vi "user.vi"() -> ()   [LabVIEW 2020]
uses:
  <userlib>/Zaphiro/GTools/Redis/Sources/Redis/Redis.lvclass/Redis.ctl
  aea59807-97c7-47ab-b578-198c3bfad1a9.vi
  f854457d-36a3-4227-beff-9843280818cc.vi
  <userlib>/Zaphiro/GTools/Redis/Sources/Redis/Connection/PING.vi
  aea59807-97c7-47ab-b578-198c3bfad1a9.vi/7c7783df-fd5a-49d9-9b7a-63cc9fb0e4e5.vi
  <userlib>/Zaphiro/GTools/Redis/Sources/Redis/Connection/QUIT.vi
  <userlib>/Zaphiro/GTools/Redis/Sources/Redis/subVIs/LL_collect-response.vi
  <userlib>/Zaphiro/GTools/Redis/Sources/Redis/Redis.lvclass
  b567c38f-e722-4316-83bf-2d80707c7bfa.vi
panel:
  out "ts":string[](array[string])
  in  "check-ts":bool
  out "meas":string[](array[string])
  in  "check-list":bool
  in  "connection":cluster{"ip":string, "port":u16, "timeout":i32}={"ip"="localhost", "port"=6379, "timeout"=1000}
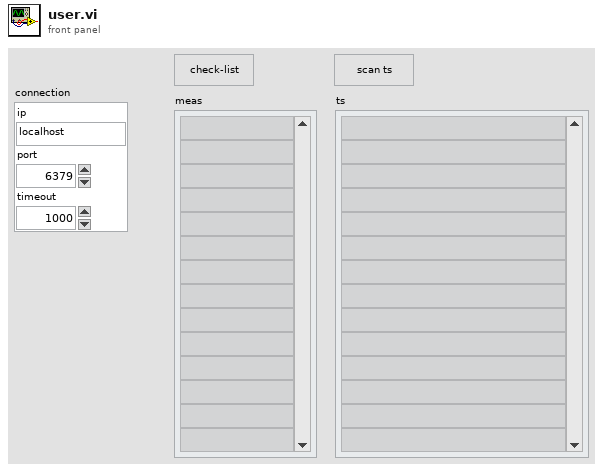
[diagram p1: front panel]
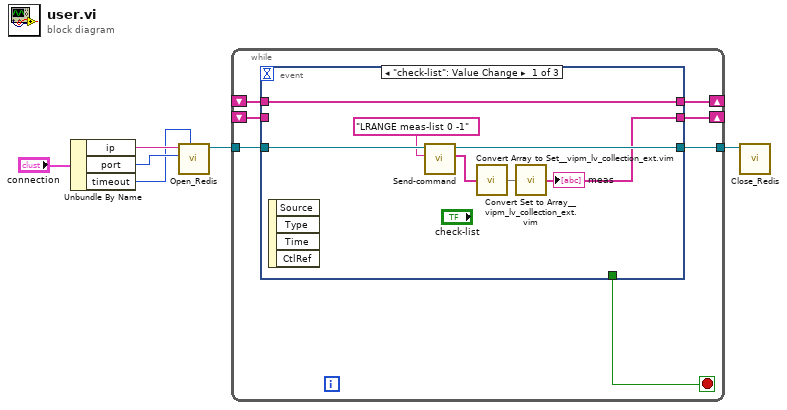
[diagram p0: block diagram]
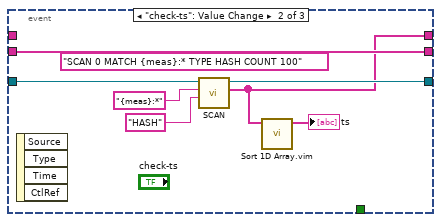
[diagram p2: hidden frame]
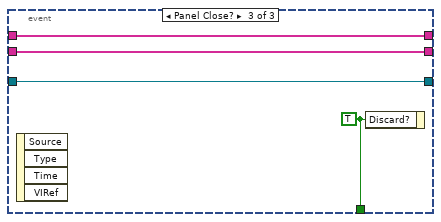
[diagram p3: hidden frame]
diagram:
  n1 = Unbundle By Name("connection") -> ("ip"=w5:string, "port"=w4:u16, "timeout"=w3:i32)
  n2 = call <userlib>:"Open_Redis.vi"("Tcp timeout ms"=w3, "Port"=w4, "Host"=w5) -> ("output cluster"=w2:refnum<class "Redis.lvclass">)  [unwired: 6 in, 2 out]
  n3 = while {
    tunnel: w2 -> [w13]
    tunnel: [w12] -> w1
    shift-right: [w10] -> _
    shift-left: _ -> [w9]
    shift-right: [w8] -> _
    shift-left: _ -> [w7]
    stop <- w11 stop-if-true
    n4 = event shown="[0] \"check-list\": Value Change" {
      selector: _ -> [_ _ _]
      dyn-events: _ -> [_ _ _]
      timeout: _ -> [_ _ _]
      tunnel: w13 -> [w20 w26 w30]
      tunnel: [w19 w25 w30] -> w12
      tunnel: [_ _ w31] -> w11
      tunnel: [w15 w27 w29] -> w10
      tunnel: w9 -> [_ w27 w29]
      tunnel: [w14 w24 w28] -> w8
      tunnel: w7 -> [w14 _ w28]
      event "check-list": Value Change {
        n5 = event-data() -> ()  [unwired: 1 in, 4 out]
        n6 = call <userlib>:"Send-command.vi"("command"="LRANGE meas-list 0 -1" ("Key"), "Redis.lvclass in"=w20) -> ("redis reply"=w16:string[], "Redis.lvclass out"=w19:refnum<class "Redis.lvclass">)  [unwired: 7 in, 1 out]
        n7 = call "Convert Array to Set__vipm_lv_collection_ext.vim"("array"=w16) -> ("set"=w17:set{string})  [unwired: 6 in]
        n8 = call "Convert Set to Array__vipm_lv_collection_ext.vim"("set"=w17) -> ("array"=w15:string[])  [unwired: 8 in]
        "meas" <- w15
      }
      event "check-ts": Value Change {
        (unwired) "SCAN 0 MATCH {meas}:* TYPE HASH COUNT 100" ("Key")
        n9 = event-data() -> ()  [unwired: 1 in, 4 out]
        n10 = call <userlib>:"SCAN.vi"("Type"="HASH" ("Key"), "Pattern"="{meas}:*" ("Key"), "Redis.lvclass in"=w26) -> ("redis reply"=w24:string[], "Redis.lvclass out"=w25:refnum<class "Redis.lvclass">)  [unwired: 6 in, 1 out]
        n11 = call "Sort 1D Array.vim"("unsorted array"=w24) -> ("sorted array"=→"ts":string[])  [unwired: 10 in]
      }
      event Panel Close? {
        w31 = TRUE ("Discard?")
        n12 = event-data() -> ()  [unwired: 1 in, 4 out]
        n13 = event-data("Discard?"=w31) -> ()  [unwired: 1 in, 1 out]
      }
    }
  }
  n14 = call <userlib>:"Close_Redis.vi"("Redis.lvclass in"=w1) -> ()  [unwired: 9 in, 2 out]
